vi "AngleMeasure.vi"(3 "error in (no error)":errorcluster, 5 "Gray Image":T2) -> (0 "error out":errorcluster, 1 "实时倾角":T1, 2 "平均倾角":dbl format="%0.2f")   [LabVIEW 2012]
uses:
  <vilib>/vision/Image Controls.llb/IMAQ Image.ctl
  <vilib>/Analysis/baseanly.llb/Unimode.vi
  <vilib>/vision/NI_Vision_Development_Module.lvlib
  <vilib>/gmath/NI_Gmath.lvlib
  <vilib>/Analysis/NI_AALBase.lvlib
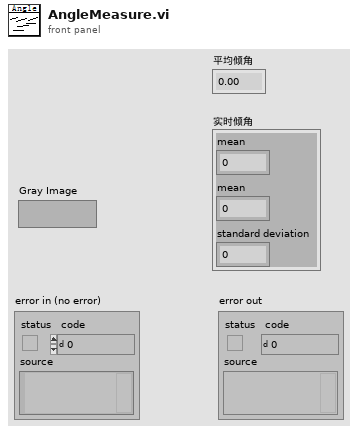
[diagram p1: front panel]
types:
  T1 = cluster{"mean":dbl, "mean":dbl, "standard deviation":dbl}
  T2 = typedef "IMAQ Image.ctl" = refnum<image>
  T3 = typedef "Particle Parameters" = i32
  T4 = cluster{"mode":dbl, "mode":dbl, "spread value":dbl}
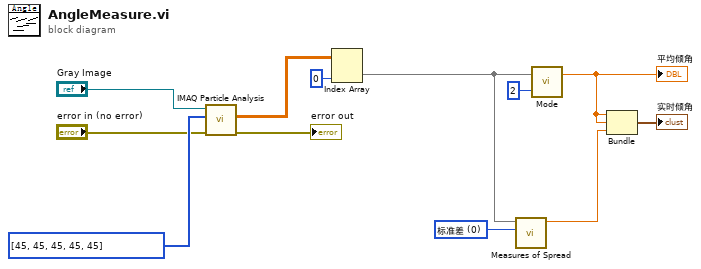
[diagram p0: block diagram]
diagram:
  w5 = 0 items=["标准差", "范围", "均值绝对偏差", "四分位数间距"] ("type")
  w12 = T3[] [45, 45, 45, 45, 45] items=["Center of Mass X", "Center of Mass Y", "First Pixel X", "First Pixel Y", "Bounding Rect Left", "Bounding Rect Top", "Bounding Rect Right", "Bounding Rect Bottom", "Max Feret Diameter Start X", "Max Feret Diameter Start Y", "Max Feret Diameter End X", "Max Feret Diameter End Y", "Max Horiz. Segment Length Left", "Max Horiz. Segment Length Right", "Max Horiz. Segment Length Row", "-", "Bounding Rect Width", "Bounding Rect Height", "Bounding Rect Diagonal", "Perimeter", "Convex Hull Perimeter", "Holes' Perimeter", "Max Feret Diameter", "Equivalent Ellipse Major Axis", "Equivalent Ellipse Minor Axis", "Equivalent Ellipse Minor Axis (Feret)", "Equivalent Rect Long Side", "Equivalent Rect Short Side", "Equivalent Rect Diagonal", "Equivalent Rect Short Side (Feret)", "Average Horiz. Segment Length", "Average Vert. Segment Length", "Hydraulic Radius", "Waddel Disk Diameter", "-", "Area", "Holes' Area", "Particle & Holes' Area", "Convex Hull Area", "Image Area", "-", "Number of Holes", "Number of Horiz. Segments", "Number of Vert. Segments", "-", "Orientation", "Max Feret Diameter Orientation", "-", "% Area/Image Area", "% Area/(Particle & Holes' Area)", "Ratio of Equivalent Ellipse Axes", "Ratio of Equivalent Rect Sides", "-", "Elongation Factor", "Compactness Factor", "Heywood Circularity Factor", "Type Factor", "-", "Sum X", "Sum Y", "Sum XX", "Sum XY", "Sum YY", "Sum XXX", "Sum XXY", "Sum XYY", "Sum YYY", "-", "Moment of Inertia XX", "Moment of Inertia XY", "Moment of Inertia YY", "Moment of Inertia XXX", "Moment of Inertia XXY", "Moment of Inertia XYY", "Moment of Inertia YYY", "Norm. Moment of Inertia XX", "Norm. Moment of Inertia XY", "Norm. Moment of Inertia YY", "Norm. Moment of Inertia XXX", "Norm. Moment of Inertia XXY", "Norm. Moment of Inertia XYY", "Norm. Moment of Inertia YYY", "Hu Moment 1", "Hu Moment 2", "Hu Moment 3", "Hu Moment 4", "Hu Moment 5", "Hu Moment 6", "Hu Moment 7"] ("Pixel Measurements")
  n1 = call "IMAQ Particle Analysis"("error in (no error)"="error in (no error)", "Pixel Measurements"=w12, "Image"="Gray Image") -> ("error out"=→"error out":errorcluster, "Particle Measurements (Pixels)"=w10:dbl[][])  [unwired: 3 in, 4 out]
  n2 = Index Array(array=w10, index (col)=0 ("禁用的索引 (列)")) -> (element=w1:dbl[])  [unwired: 1 in]
  n3 = call <vilib>:"Measures of Spread.vi"("type"=w5, "x array"=w1) -> ("spread value"=w2:dbl)  [unwired: 8 in, 1 out]
  n4 = call-poly <vilib>:"Mode.vi"("intervals"=2, "X"=w1) -> ("mode"=w3:dbl)  [unwired: 1 out]
  "平均倾角" <- w3
  n5 = Bundle("mode"=w3, "mode"=w3, "spread value"=w2) -> (→"实时倾角":T4)  [unwired: 1 in]
